vi "单线性拉伸曲线图.vi"(2 "数组－数值 2":dbl[](array[numeric]), 3 "数组－数值":dbl[](array[numeric])) -> (0 "弯曲刚度值":dbl, 1 "XY Graph":cluster{"Y":dbl[], "Y":dbl[]}[](graph) caption="弯曲刚度")   [LabVIEW 2016]
uses:
  <vilib>/Analysis/NI_AALPro.lvlib
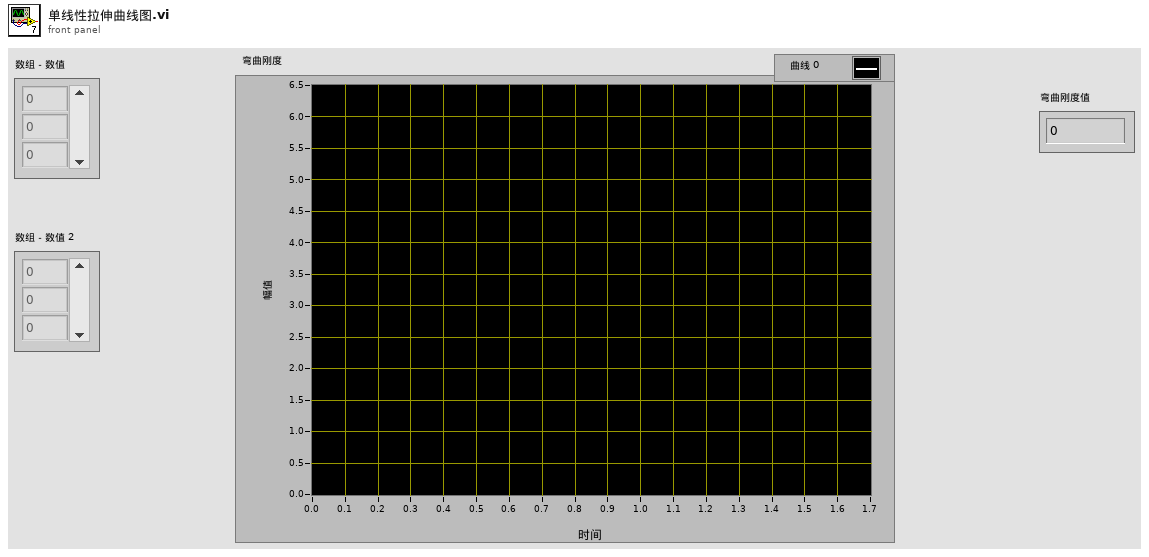
[diagram p1: front panel]
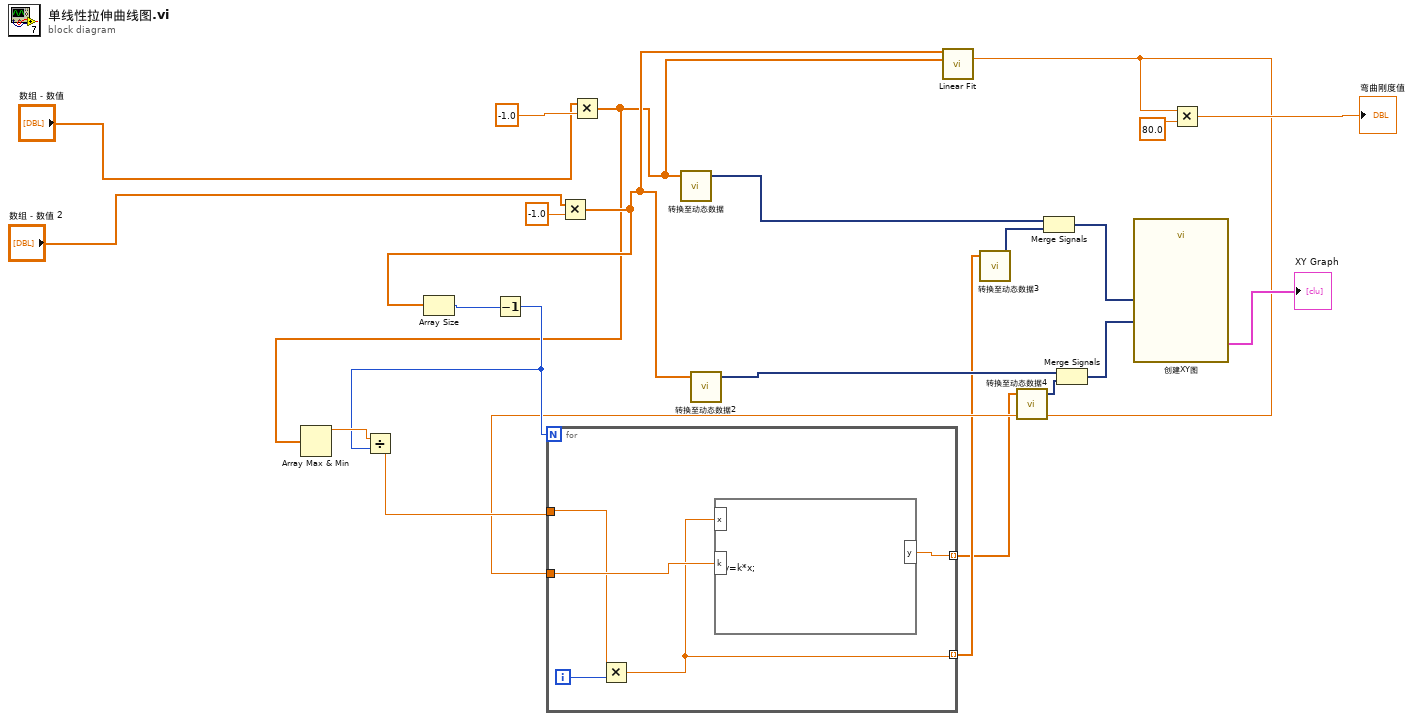
[diagram p0: block diagram]
diagram:
  n1 = Multiply(x="数组－数值 2", y=-1.0) -> (x*y=w6:dbl[])
  n2 = Array Size(array=w6) -> (size(s)=w17:i32)
  n3 = Decrement(x=w17) -> (x-1=w15:i32)
  n4 = Multiply(x="数组－数值", y=-1.0) -> (x*y=w3:dbl[])
  n5 = Array Max & Min(array=w3) -> (max value=w16:dbl)  [unwired: 3 out]
  n6 = Divide(x=w16, y=w15) -> (x/y=w14:dbl)
  n7 = call "转换至动态数据"("Array"=w3) -> ("Dynamic Data Type"=w22:dynamicdata)  [unwired: 3 in]
  n8 = call "转换至动态数据2"("Array"=w6) -> ("Dynamic Data Type"=w21:dynamicdata)  [unwired: 3 in]
  n9 = call <vilib>:"Linear Fit.vi"("Y"=w6, "X"=w3) -> ("slope"=w7:dbl)  [unwired: 9 in, 4 out]
  n10 = for {
    N: w15 -> [_]
    tunnel: w7 -> [w27]
    tunnel: [w26] -> w4 mode=indexing
    tunnel: [w23] -> w5 mode=indexing
    tunnel: w14 -> [w25]
    i -> [w24]
    n11 = Multiply(x=w25, y=w24) -> (x*y=w23:dbl)
    n12 = formula code="y=k*x;"("x"=w23, "k"=w27) -> ("y"=w26:dbl)
  }
  n13 = call "转换至动态数据3"("Array"=w5) -> ("Dynamic Data Type"=w13:dynamicdata)  [unwired: 3 in]
  n14 = call "转换至动态数据4"("Array"=w4) -> ("Dynamic Data Type"=w12:dynamicdata)  [unwired: 3 in]
  n15 = Merge Signals(w22, w13) -> (w20:dynamicdata)
  n16 = Merge Signals(w21, w12) -> (w19:dynamicdata)
  n17 = call "创建XY图"("Y Input"=w19, "X Input"=w20) -> ("XY Graph"=→"XY Graph":cluster{"X":dbl[], "Y":dbl[]}[])  [unwired: 8 in, 1 out]
  n18 = Multiply(x=w7, y=80.0) -> (x*y=→"弯曲刚度值":dbl)
